vi "DCAM_sub_vi_configure_ouput_triggers.vi"(3 "error in (no error)":errorcluster, 5 "Handle in":u32) -> (0 "error out":errorcluster, 2 "Handle out":u32)   [LabVIEW 2015]
panel:
  # "Configure Output Triggers:  Common for all of my use cases."
  # "This VI just cleans up some clutter (for practice)"
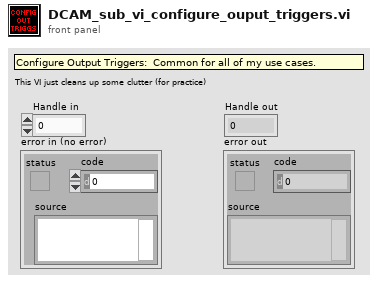
[diagram p1: front panel]
types:
  T1 = cluster{"Mode":u32, "Polarity":u32, "Period":dbl, "Delay":dbl}
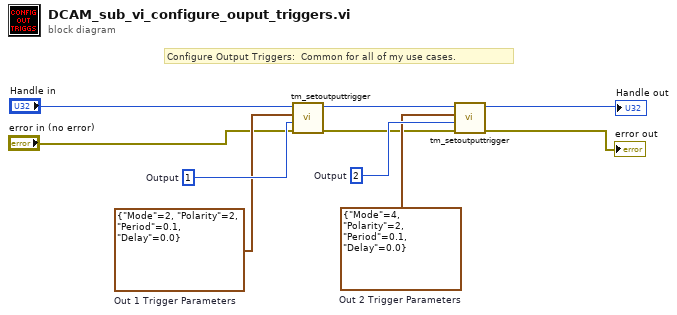
[diagram p0: block diagram]
diagram:
  w7 = T1 {"Mode"=4, "Polarity"=2, "Period"=0.1, "Delay"=0.0}  # Out 2 Trigger Parameters
  w8 = T1 {"Mode"=2, "Polarity"=2, "Period"=0.1, "Delay"=0.0}  # Out 1 Trigger Parameters
  w9 = 2  # Output
  w10 = 1  # Output
  # "Configure Output Triggers:  Common for all of my use cases."
  n1 = call <userlib>:"tm_setoutputtrigger.vi"("error in (no error)"="error in (no error)", "Index"=w10, "Parameters"=w8, "Handle in"="Handle in") -> ("error out"=w6:errorcluster, "Handle out"=w5:u32)  [unwired: 6 in]
  n2 = call <userlib>:"tm_setoutputtrigger.vi"("error in (no error)"=w6, "Index"=w9, "Parameters"=w7, "Handle in"=w5) -> ("error out"=→"error out":errorcluster, "Handle out"=→"Handle out":u32)  [unwired: 6 in]
